vi "PH_uOPA_DelayController.Action Get data.vi"(0 "i ref in":refnum<vi>, 5 "error IO":errorcluster) -> (14 "i ref out":refnum<vi>, 19 "error out":errorcluster)   [LabVIEW 2014, in "PH_uOPA_DelayController.lvlib"]
doc: "This is the action within the proc case \"Get Data\": The data are analysied and indicated."
uses:
  PH_uOPA_DelayController.lvlib
  PH_Basics/PH_AxisGUI_BaseClass/PH_AxisGUI_BaseClass.lvlib
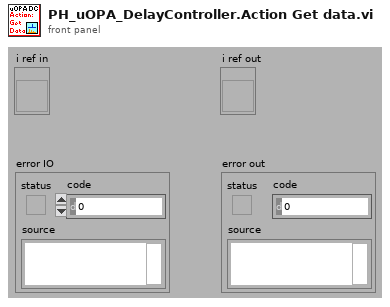
[diagram p1: front panel]
types:
  T1 = typedef "PH_AxisGUI_BaseClass.lvlib/PH_AxisGUI_BaseClass.i attribute.ctl" = cluster{"Axes":T2[]}
  T2 = typedef "PH_AxisGUI_BaseClass.lvlib/PH_AxisGUI_BaseClass.Axis Attributes.ctl" = cluster{"Axis GUI Refs":T3, "Address":T4, "Name":string, "Label \"Back\"":string, "Labell \"Forth\"":string, "Moving?":bool}
  T3 = typedef "PH_AxisGUI_BaseClass.lvlib/PH_AxisGUI_BaseClass.Axis GUI Refs.ctl" = cluster{"Back":refnum<vi>, "Forth":refnum<vi>, "Status":refnum<vi>, "Target":refnum<vi>, "Address":refnum<vi>, "Status Bar":refnum<vi>, "Settings":refnum<vi>, "Activity":refnum<vi>, "Clear Error":refnum<vi>}
  T4 = typedef "PH_Stepmotor_BaseClass.lvlib/PH_Stepmotor_BaseClass.Axis Address.ctl" = cluster{"Instance":string, "Motor Nr":i32}
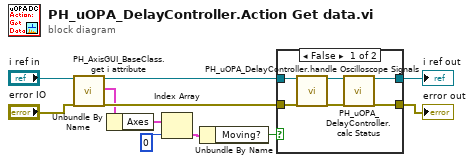
[diagram p0: block diagram]
diagram:
  n1 = call "PH_AxisGUI_BaseClass.get i attribute.vi"("i ref in"="i ref in", "error in (no error)"="error IO") -> ("i ref out"=w6:refnum<vi>, "i attribute"=w5:T1, "error out"=w8:errorcluster)  [unwired: 15 in]
  n2 = Unbundle By Name(w5) -> ("Axes"=w4:T2[])
  n3 = Index Array(array=w4, index=0) -> (element=w2:T2)
  n4 = Unbundle By Name(w2) -> ("Moving?"=w1:bool)
  n5 = case shown="False" w1 {
    tunnel: [w14 w19] -> w11
    tunnel: [w15 w18] -> w10
    tunnel: w8 -> [w17 w18]
    tunnel: w6 -> [w16 w19]
    frame False {
      n6 = call "PH_uOPA_DelayController.handle Oscilloscope Signals.vi"("VI in"=w16, "error in"=w17) -> ("VI out"=w13:refnum<vi>, "error out"=w12:errorcluster)  [unwired: 16 in]
      n7 = call "PH_uOPA_DelayController.calc Status.vi"("i ref in"=w13, "error in"=w12) -> ("i ref out"=w14:refnum<vi>, "error out"=w15:errorcluster)  [unwired: 16 in]
    }
    frame True {
    }
  }
  "error out" <- w10
  "i ref out" <- w11
